vi "ReadAgilent53131A_DL_mk2.VI"(1 "GPIB address":string="10") -> (0 "[MHz]":dbl=100.000124 format="%#_10g")   [LabVIEW 2021]
panel:
  in  "Desired measurement number":i32
  out "Measurement number":i32
  out "Waveform Chart":dbl(graph)
  out "Decoded output":dbl=100000124.0
  out "OUTPUT":string="+1.00000124E+008\n"
  in  "byte count":i32=38
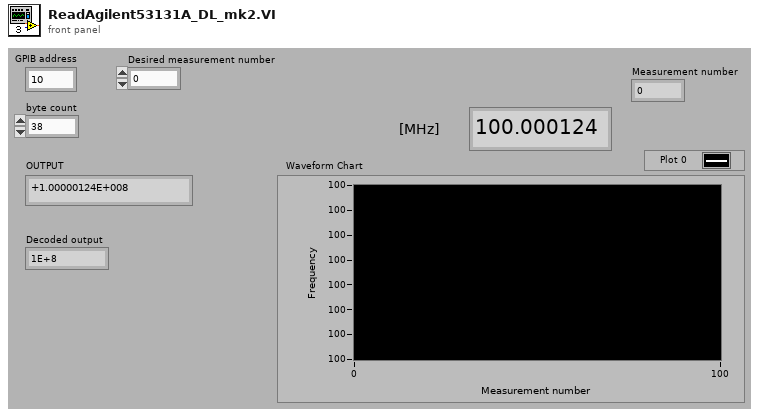
[diagram p1: front panel]
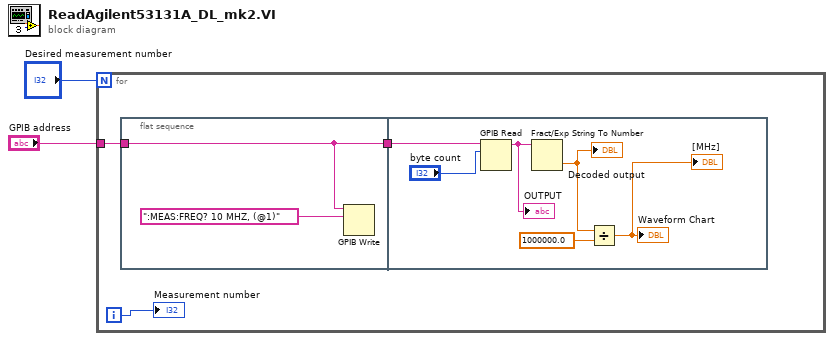
[diagram p0: block diagram]
diagram:
  n1 = for {
    N: "Desired measurement number" -> [_]
    tunnel: "GPIB address" -> [w4]
    i -> [w3]
    n2 = flat-sequence {
      tunnel: w4 -> [w7]
      tunnel: [w7] -> w5
      tunnel: w5 -> [w13]
      frame #0 {
        n3 = GPIB Write(0:w7, 1:":MEAS:FREQ? 10 MHZ, (@1)" ("polecenie")) -> ()  [unwired: 3 in, 2 out]
      }
      frame #1 {
        n4 = GPIB Read(0:w13, 1:"byte count") -> (5:w10:string)  [unwired: 3 in, 2 out]
        "OUTPUT" <- w10
        n5 = Fract/Exp String To Number(string=w10) -> (number=w11:dbl)  [unwired: 3 in, 1 out]
        "Decoded output" <- w11
        n6 = Divide(x=w11, y=1000000.0) -> (x/y=→"[MHz]" →"Waveform Chart":dbl)
      }
    }
    "Measurement number" <- w3
  }
